vi "Config Measure Settings.vi"(0 "VISA resource name":refnum<visa-resource-name>, 1 "Autozero (Auto)":enum32{"Off", "Once", "Auto"}(ring)=enum."Auto", 2 "Sense (2 Wire)":enum32{"2 Wire", "4 Wire", "Calibration"}(ring), 3 "NPLC (1.000)":dbl=1.0, 5 "Node In":string, 7 "Channel (Channel A)":T1, 9 "Measure Delay (0)":dbl, 11 "error in":errorcluster, 12 "Measure Count (1)":u32=1, 13 "Interval (0.000)":dbl) -> (4 "VISA resource name out":refnum<visa-resource-name>, 6 "Node Out":string, 14 "Command String":string, 15 "error out":errorcluster)   [LabVIEW 2018, in "Keithley 2600 Series.lvlib"]
doc: "This VI configures general measurement settings that apply to all measure functions.\n\n<b>Note:</b> This VI does not configure the measurement filter. Please use Configure Measure Filter to configure the filter.\n\n<b>Functions and Attributes Used</b>\nsmuX.measure.count\nsmuX.measure.interval\nsmuX.measure.nplc"
uses:
  Keithley 2600 Series.lvlib
  Private/GlobalVariables.vi
  Channel.ctl
panel:
  # "(c) 2008 Keithley Instruments, Inc.  ALL RIGHTS RESERVED."
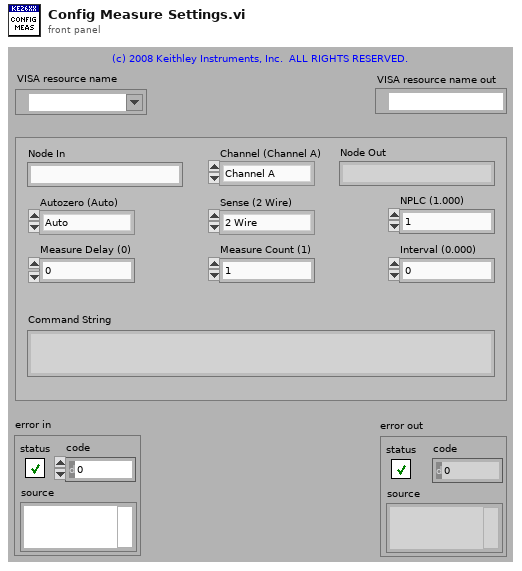
[diagram p1: front panel]
types:
  T1 = typedef "Keithley 2600 Series.lvlib/Channel.ctl" = enum32{"Channel A", "Channel B"}
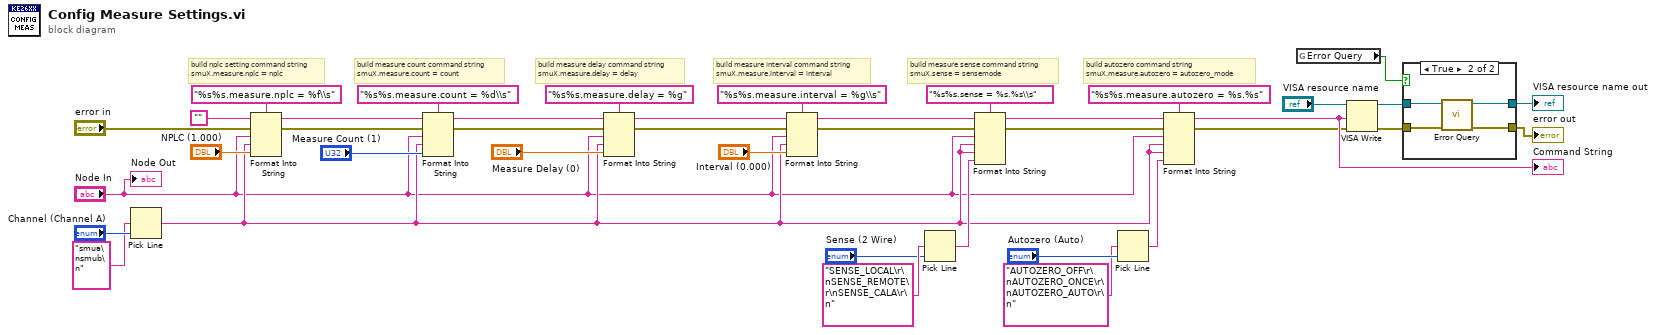
[diagram p0: block diagram]
diagram:
  # "build measure delay command string\nsmuX.measure.delay = delay"
  # "build autozero command string\nsmuX.measure.autozero = autozero_mode"
  # "build measure sense command string\nsmuX.sense = sensemode"
  # "build measure interval command string\nsmuX.measure.interval = interval"
  # "build measure count command string\nsmuX.measure.count = count"
  # "build nplc setting command string\nsmuX.measure.nplc = nplc"
  n1 = Pick Line(multi-line string="smua\nsmub\n", line index="Channel (Channel A)") -> (output string=w2:string)  [unwired: 1 out]
  n2 = Format Into String(format string="%s%s.measure.nplc = %f\\s", initial string="", error in="error in", "Node In", w2, "NPLC (1.000)") -> (resulting string=w32:string, error out=w31:errorcluster)
  n3 = Format Into String(format string="%s%s.measure.count = %d\\s", initial string=w32, error in=w31, "Node In", w2, "Measure Count (1)") -> (resulting string=w8:string, error out=w7:errorcluster)
  n4 = Format Into String(format string="%s%s.measure.delay = %g", initial string=w8, error in=w7, "Node In", w2, "Measure Delay (0)") -> (resulting string=w5:string, error out=w6:errorcluster)
  n5 = Format Into String(format string="%s%s.measure.interval = %g\\s", initial string=w5, error in=w6, "Node In", w2, "Interval (0.000)") -> (resulting string=w16:string, error out=w15:errorcluster)
  n6 = Pick Line(multi-line string="SENSE_LOCAL\r\nSENSE_REMOTE\r\nSENSE_CALA\r\n" ("options"), line index="Sense (2 Wire)") -> (output string=w12:string)  [unwired: 1 out]
  n7 = Format Into String(format string="%s%s.sense = %s.%s\\s", initial string=w16, error in=w15, "Node In", w2, w2, w12) -> (resulting string=w14:string, error out=w13:errorcluster)
  n8 = Pick Line(multi-line string="AUTOZERO_OFF\r\nAUTOZERO_ONCE\r\nAUTOZERO_AUTO\r\n" ("options"), line index="Autozero (Auto)") -> (output string=w11:string)  [unwired: 1 out]
  n9 = Format Into String(format string="%s%s.measure.autozero = %s.%s", initial string=w14, error in=w13, "Node In", w2, w2, w11) -> (resulting string=w10:string, error out=w9:errorcluster)
  "Command String" <- w10
  n10 = global read "GlobalVariables.vi" "Error Query"() -> (w25:bool)
  n11 = VISA Write(VISA resource name="VISA resource name", write buffer=w10, error in (no error)=w9) -> (VISA resource name out=w27:refnum<visa-resource-name>, error out=w26:errorcluster)  [unwired: 1 out]
  n12 = case shown="True" w25 {
    tunnel: w27 -> [w42 w46]
    tunnel: w26 -> [w41 w45]
    tunnel: [w42 w44] -> w24
    tunnel: [w41 w43] -> w23
    frame False {
    }
    frame True {
      n13 = call "Error Query.vi"("error in (no error)"=w45, "VISA resource name"=w46) -> ("error out"=w43:errorcluster, "VISA resource name out"=w44:refnum<visa-resource-name>)  [unwired: 8 out]
    }
  }
  "VISA resource name out" <- w24
  "error out" <- w23
  "Node Out" <- "Node In"
